vi "Unflatten-WindowEventData.vi"(8 "error in (no error)":errorcluster, 11 "Event Binary Data":string) -> (0 "error out":errorcluster, 3 "WindowEvent":T1)   [LabVIEW 2026, in "SDL3.lvlib" / "Events.lvlib"]
uses:
  Video/WindowID--integer.ctl
  Events.lvlib
  Video/Video.lvlib
  WindowEvent--cluster.ctl
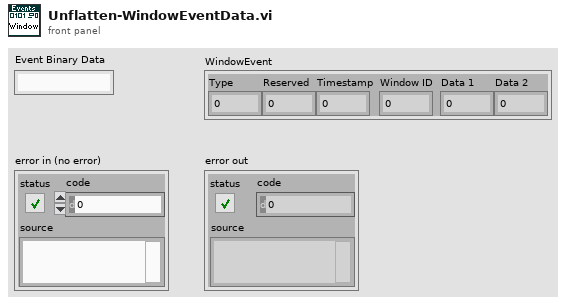
[diagram p1: front panel]
types:
  T1 = typedef "SDL3.lvlib/Events.lvlib/WindowEvent--cluster.ctl" = cluster{"Type":u32, "Reserved":u32, "Timestamp":u64, "Window ID":T2, "Data 1":i32, "Data 2":i32}
  T2 = typedef "SDL3.lvlib/Video.lvlib/WindowID--integer.ctl" = u32
  T3 = enum16{"big-endian, network order", "native, host order", "little-endian"}
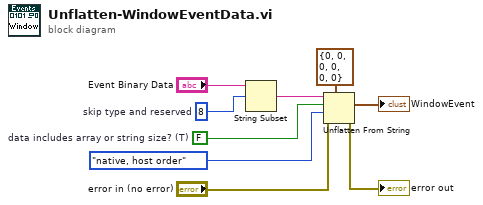
[diagram p0: block diagram]
diagram:
  w3 = 8  # skip type and reserved
  w6 = FALSE  # data includes array or string size? (T)
  n1 = String Subset(string="Event Binary Data", offset (0)=w3) -> (substring=w4:string)  [unwired: 1 in]
  n2 = Unflatten From String(type=T1 {"Type"=0, "Reserved"=0, "Timestamp"=0, "Window ID"=0, "Data 1"=0, "Data 2"=0} ("WindowEvent"), binary string=w4, data includes array or string size? (T)=w6, byte order (0:big-endian, network order)=T3."native, host order", error in (no error)="error in (no error)") -> (value=→"WindowEvent":T1, error out=→"error out":errorcluster)  [unwired: 1 out]
